vi "InitValves.vi"   [LabVIEW 2013]
uses:
  GlobalVariables/ValveValues.vi
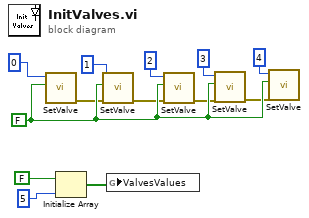
[diagram p0: block diagram]
diagram:
  w10 = FALSE
  n1 = call "SetValve.vi"("ON"=w10, "Valve"=u16 0) -> ("error out"=w9:errorcluster)  [unwired: 9 in]
  n2 = Initialize Array(FALSE, 5) -> (w11:bool[])
  n3 = call "SetValve.vi"("error in"=w9, "ON"=w10, "Valve"=u16 1) -> ("error out"=w8:errorcluster)  [unwired: 8 in]
  n4 = global write "ValveValues.vi" "ValvesValues"(w11) -> ()
  n5 = call "SetValve.vi"("error in"=w8, "ON"=w10, "Valve"=u16 2) -> ("error out"=w7:errorcluster)  [unwired: 8 in]
  n6 = call "SetValve.vi"("error in"=w7, "ON"=w10, "Valve"=u16 3) -> ("error out"=w6:errorcluster)  [unwired: 8 in]
  n7 = call "SetValve.vi"("error in"=w6, "ON"=w10, "Valve"=u16 4) -> ()  [unwired: 8 in, 1 out]
